vi "Query Ambient Temperature.vi"(8 "error in (no error)":errorcluster, 11 "VISA resource name":refnum<visa-resource-name>) -> (0 "error out":errorcluster, 1 "Timestamp":string, 2 "Temperature":dbl format="%^.3e", 3 "VISA resource name out":refnum<visa-resource-name>, 4 "Box":string)   [LabVIEW 2020, in "Rohde&Schwarz CMXP Base.lvlib"]
doc: "Queries the ambient temperature measured via a sensor in the instrument.\n\nAmbient temperatures reported by self-tests are also measured via this sensor.\n\nAttribute:\n-\n\nRemote-control command:\nSENSe:BASE:TEMPerature:OPERating:AMBient?"
uses:
  <instrlib>/Rohde&Schwarz CMXP Base/Rohde&Schwarz CMXP Base.lvlib
  <instrlib>/Rohde&Schwarz CMXP Base/Private/rsidr_core.llb/rsidr_core.lvlib
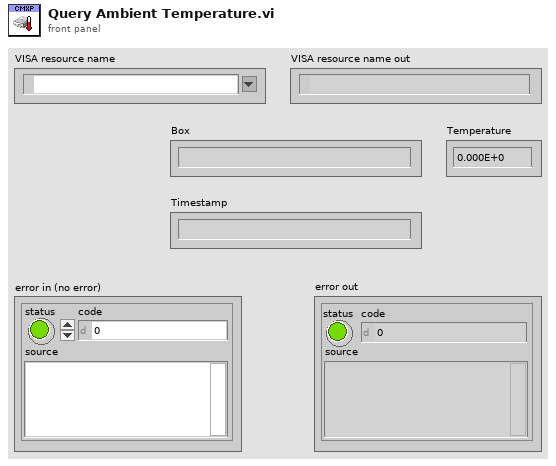
[diagram p1: front panel]
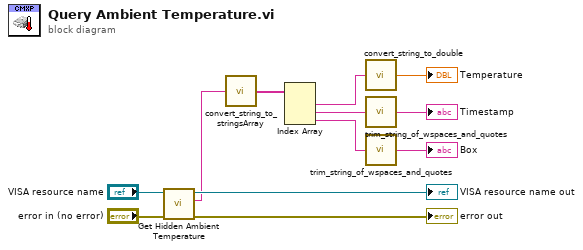
[diagram p0: block diagram]
diagram:
  n1 = call "Get Hidden Ambient Temperature"("error in (no error)"="error in (no error)", "instrument handle"="VISA resource name") -> ("error out"=→"error out":errorcluster, "Hidden Ambient Temperature"=w3:string, "instrument handle out"=→"VISA resource name out":refnum<visa-resource-name>)  [unwired: 7 in]
  n2 = call <instrlib>:"convert_string_to_stringsArray.vi"("String in"=w3) -> ("string array out"=w7:string[])  [unwired: 3 in, 1 out]
  n3 = Index Array(array=w7) -> (element #1=w2:string, element #2=w6:string, element #3=w1:string)  [unwired: 3 in]
  n4 = call <instrlib>:"convert_string_to_double.vi"("String in"=w2) -> ("double value out"=→"Temperature":dbl)  [unwired: 4 in]
  n5 = call <instrlib>:"trim_string_of_wspaces_and_quotes.vi"("String in"=w6) -> ("String out"=→"Timestamp":string)  [unwired: 4 in]
  n6 = call <instrlib>:"trim_string_of_wspaces_and_quotes.vi"("String in"=w1) -> ("String out"=→"Box":string)  [unwired: 4 in]
